vi "4 - Analysis and Output (Solution).vi"() -> ()   [LabVIEW 2012]
panel:
  out "Alarm Output":bool
  in  "Alarm Level":dbl=26.0
  out "Temperature Data":dynamicdata(graph)
  in  "stop":bool
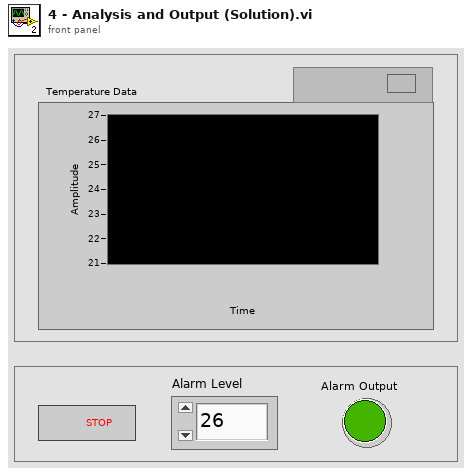
[diagram p1: front panel]
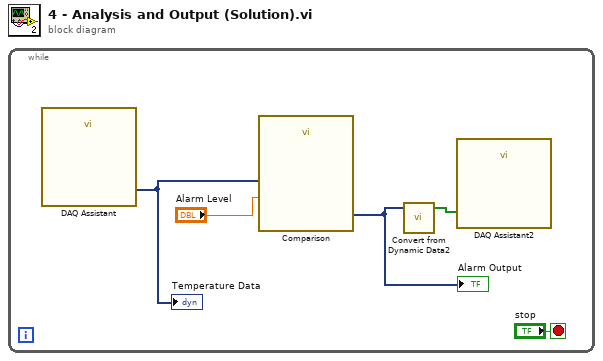
[diagram p0: block diagram]
diagram:
  n1 = while {
    stop <- "stop" stop-if-true
    n2 = call "DAQ Assistant"() -> ("data"=w1:dynamicdata)  [unwired: 16 in, 3 out]
    "Temperature Data" <- w1
    n3 = call "Comparison"("Operand 2"="Alarm Level", "Operand 1"=w1) -> ("Result"=w2:dynamicdata)  [unwired: 1 in, 8 out]
    "Alarm Output" <- w2
    n4 = call "Convert from Dynamic Data2"("Dynamic Data Type"=w2) -> ("Array"=w3:bool[])  [unwired: 3 out]
    n5 = call "DAQ Assistant2"("data"=w3) -> ()  [unwired: 4 in, 15 out]
  }
